vi "Drive For Angle Controller.vi"(8 "Vision":bool, 9 "Speed":dbl, 10 "Yaw":dbl, 11 "Iterations":i32) -> (1 "Right Setpoint":dbl, 2 "Left Setpoint":dbl, 3 "Finished?":bool)   [LabVIEW 2016]
uses:
  <vilib>/Rock Robotics/Network Tables/NT Read Number.vi
  NavX/NavX Global.vi
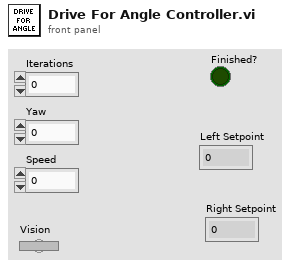
[diagram p1: front panel]
types:
  T1 = cluster{"Yaw":dbl, "Roll":dbl, "Pitch":dbl, "Heading":dbl, "Fused Heading":dbl}
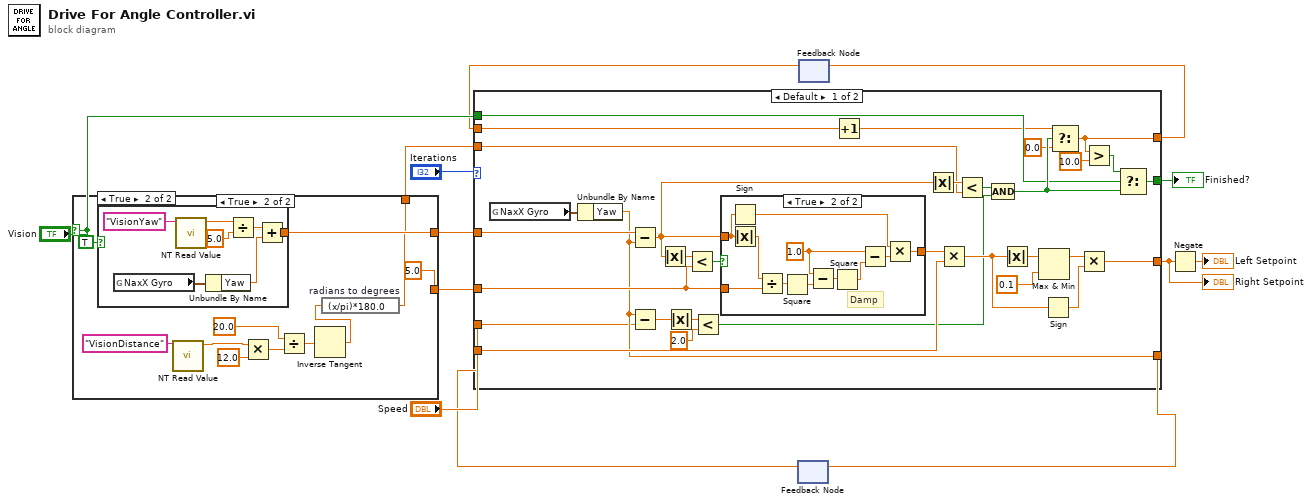
[diagram p0: block diagram]
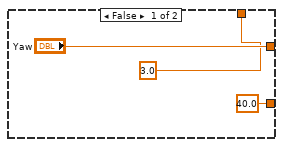
[diagram p2: hidden frame]
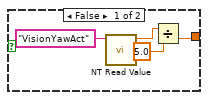
[diagram p3: hidden frame]
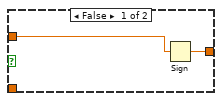
[diagram p4: hidden frame]
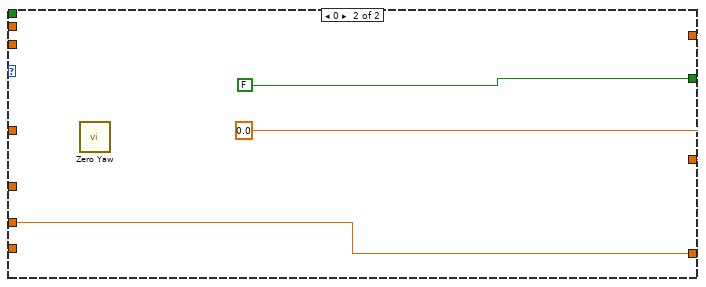
[diagram p5: hidden frame]
diagram:
  n1 = case shown="True" "Vision" {
    tunnel: ["Yaw" w27] -> w12
    tunnel: [3.0 ("y") w17] -> w2
    tunnel: [40.0 5.0] -> w1
    frame False {
    }
    frame True {
      n2 = case shown="True" TRUE {
        tunnel: [w30 w36] -> w27
        frame False {
          n3 = call-poly <vilib>:"NT Read Value.vi"("Name"="VisionYawAct") -> ("Numeric"=w29:dbl)  [unwired: 9 in, 1 out]
          n4 = Divide(x=w29, y=5.0) -> (x/y=w30:dbl)
        }
        frame True {
          n5 = global read "NavX Global.vi" "NaxX Gyro"() -> (w37:T1)
          n6 = call-poly <vilib>:"NT Read Value.vi"("Name"="VisionYaw") -> ("Numeric"=w34:dbl)  [unwired: 9 in, 1 out]
          n7 = Unbundle By Name(w37) -> ("Yaw"=w35:dbl)
          n8 = Divide(x=w34, y=5.0) -> (x/y=w33:dbl)
          n9 = Add(x=w33, y=w35) -> (x+y=w36:dbl)
        }
      }
      n10 = call-poly <vilib>:"NT Read Value.vi"("Name"="VisionDistance") -> ("Numeric"=w23:dbl)  [unwired: 9 in, 1 out]
      n11 = Multiply(x=w23, y=12.0) -> (x*y=w22:dbl)
      n12 = Divide(x=20.0, y=w22) -> (x/y=w20:dbl)
      n13 = Inverse Tangent(1:w20) -> (0:w19:dbl)
      n14 = expression code="(x/pi)*180.0" "radians to degrees"(w19) -> (w17:dbl)
    }
  }
  n15 = feedback #1() -> (w6:dbl)  [unwired: 1 in]
  n16 = feedback #2() -> (w4:dbl)  [unwired: 1 in]
  n17 = case shown="Default" "Iterations" {
    tunnel: w12 -> [w68 _]
    tunnel: "Speed" -> [w69 _]
    tunnel: [w61 w84] -> w8
    tunnel: [w50 FALSE] -> w10
    tunnel: w1 -> [w57 _]
    tunnel: [w55 w85] -> w7
    tunnel: w6 -> [w54 w85]
    tunnel: "Vision" -> [w43 _]
    tunnel: [w47 w84] -> w3
    tunnel: w4 -> [w45 _]
    tunnel: w2 -> [w39 _]
    frame Default {
      n18 = global read "NavX Global.vi" "NaxX Gyro"() -> (w70:T1)
      n19 = Unbundle By Name(w70) -> ("Yaw"=w55:dbl)
      n20 = Subtract(x=w68, y=w55) -> (x-y=w60:dbl)
      n21 = Subtract(x=w55, y=w54) -> (x-y=w51:dbl)
      n22 = Absolute Value(x=w60) -> (abs(x)=w58:dbl)
      n23 = Absolute Value(x=w51) -> (abs(x)=w52:dbl)
      n24 = Less?(x=w58, y=w57) -> (x < y?=w59:bool)
      n25 = Less?(x=w52, y=2.0) -> (x < y?=w41:bool)
      n26 = case shown="True" w59 {
        tunnel: w60 -> [w71 w77]
        tunnel: w57 -> [_ w80]
        tunnel: [w72 w75] -> w65
        frame False {
          n27 = Sign(1:w71) -> (0:w72:dbl)
        }
        frame True {
          w81 = 1.0
          # "Damp"
          n28 = Sign(1:w77) -> (0:w74:dbl)
          n29 = Absolute Value(x=w77) -> (abs(x)=w78:dbl)
          n30 = Divide(x=w78, y=w80) -> (x/y=w79:dbl)
          n31 = Square(x=w79) -> (x^2=w83:dbl)
          n32 = Subtract(x=w81, y=w83) -> (x-y=w82:dbl)
          n33 = Square(x=w82) -> (x^2=w73:dbl)
          n34 = Subtract(x=w81, y=w73) -> (x-y=w76:dbl)
          n35 = Multiply(x=w74, y=w76) -> (x*y=w75:dbl)
        }
      }
      n36 = Increment(x=w45) -> (x+1=w42:dbl)
      n37 = Absolute Value(x=w60) -> (abs(x)=w67:dbl)
      n38 = Multiply(x=w65, y=w69) -> (x*y=w56:dbl)
      n39 = Less?(x=w67, y=w39) -> (x < y?=w66:bool)
      n40 = Compound Arithmetic op=AND(w66, w41) -> (w49:bool)
      n41 = Absolute Value(x=w56) -> (abs(x)=w64:dbl)
      n42 = Max & Min(x=w64, y=0.1) -> (max(x,y)=w63:dbl)  [unwired: 1 out]
      n43 = Sign(1:w56) -> (0:w62:dbl)
      n44 = Select(t=w42, s=w49, f=0.0) -> (s? t:f=w47:dbl)
      n45 = Multiply(x=w63, y=w62) -> (x*y=w61:dbl)
      n46 = Greater?(x=w47, y=10.0) -> (0:w48:bool)
      n47 = Select(t=w48, s=w43, f=w49) -> (s? t:f=w50:bool)
    }
    frame 0 {
      w84 = 0.0
      n48 = call <vilib>:"Zero Yaw.vi"() -> ()  [unwired: 12 in]
    }
  }
  "Finished?" <- w10
  "Right Setpoint" <- w8
  n49 = feedback-in #1(w7) -> ()
  n50 = feedback-in #2(w3) -> ()
  n51 = Negate(x=w8) -> (-x=→"Left Setpoint":dbl)
